vi "PicoScope5000aSetDataBuffers.vi"(5 "enabled array":i16[](array[numeric]), 7 "Buffer and Transfer Settings":T3={"startIndex"=0, "Samples"=1000, "Down Sample Ratio"=1, "Down-Sample Mode"=1} {"Down-Sample Mode" items=["RAW none"=2147483648, "None"=0, "Aggregate"=1, "Decimate"=2, "Average"=4]; "Down Sample Ratio" step=1; "Samples" format="%_6p"}, 8 "error in (no error)":errorcluster, 9 "Device Info":T1={"Driver Version"="2.1.104.3324", "USB Version"="2.0", "Hardware"="1", "Variant"="5244A", "Batch and Serial"="CQ178/007", "Cal Date"="11Jun13", "Kernel Version"="1.0", "Digital HW Version"="1", "Analogue HW Version"="1", "MSO"=FALSE, "Number of channels"=2}, 10 "Data Pointers In":T2, 11 "handle in":i16) -> (0 "error out":errorcluster, 3 "handle out":i16)   [LabVIEW 2010]
doc: "Calls ps5000aSetDataBuffers, and assigns Pico buffers"
uses:
  ps5000a.dll
  shared/PicoBuffers.ctl
  shared/Buffer and Transfer Settings.ctl
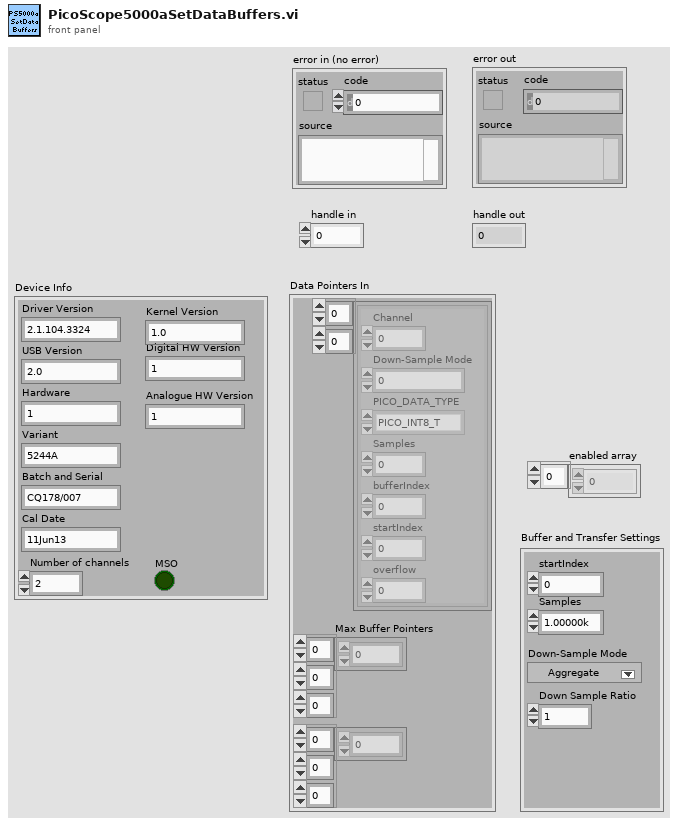
[diagram p1: front panel]
types:
  T1 = cluster{"Driver Version":string, "USB Version":string, "Hardware":string, "Variant":string, "Batch and Serial":string, "Cal Date":string, "Kernel Version":string, "Digital HW Version":string, "Analogue HW Version":string, "MSO":bool, "Number of channels":i16}
  T2 = typedef "PicoBuffers.ctl" = cluster{"Max Buffer Pointers":u64[][][], "Min Buffer Pointers":u64[][][], "StreamingDataInfo":cluster{"Channel":u32, "Down-Sample Mode":u32, "PICO_DATA_TYPE":enum32{"PICO_INT8_T", "PICO_INT16_T", "PICO_INT32_T", "PICO_UINT32_T", "PICO_INT64_T", ""}, "Samples":i32, "bufferIndex":u64, "startIndex":i32, "overflow":i16}[][]}
  T3 = typedef "Buffer and Transfer Settings.ctl" = cluster{"startIndex":u64, "Samples":u64, "Down Sample Ratio":u64, "Down-Sample Mode":u32}
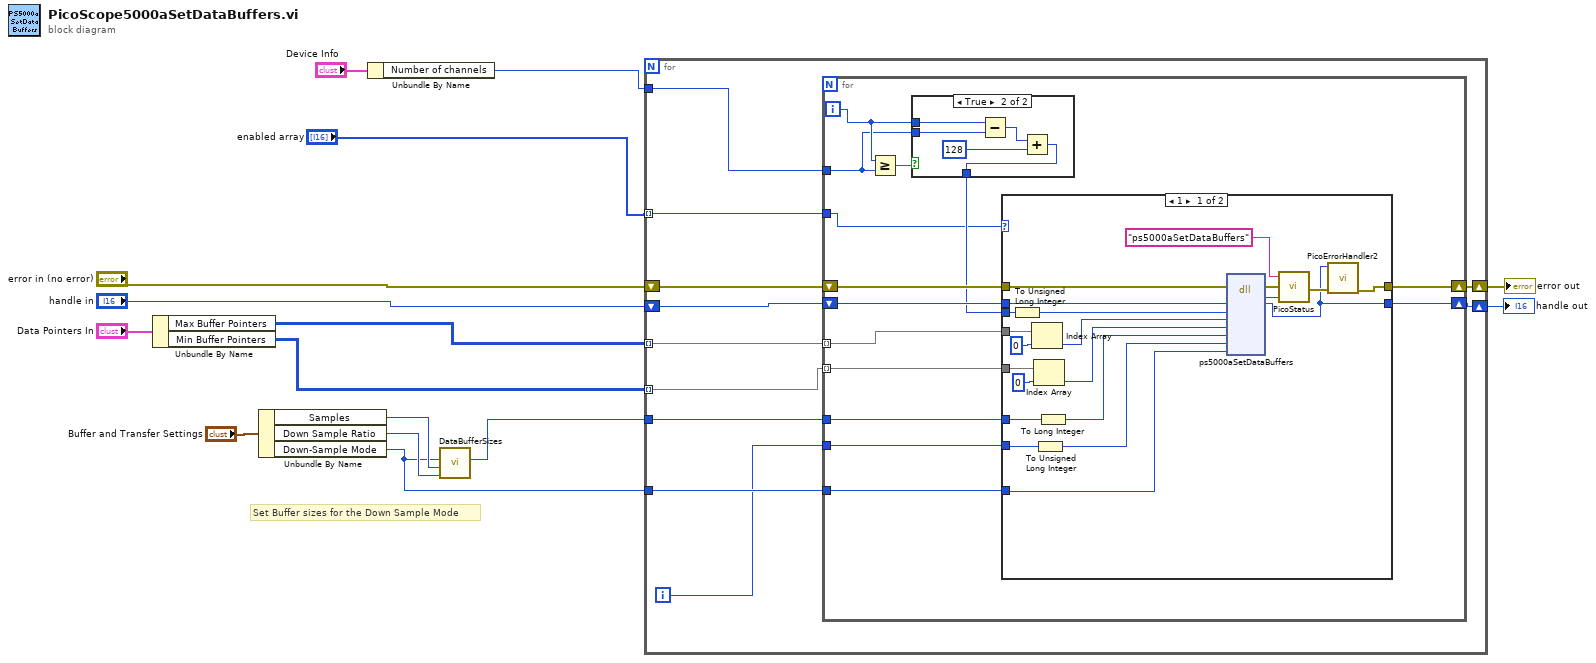
[diagram p0: block diagram]
diagram:
  # "Set Buffer sizes for the Down Sample Mode"
  n1 = Unbundle By Name("Data Pointers In") -> ("Max Buffer Pointers"=w7:u64[][][], "Min Buffer Pointers"=w6:u64[][][])
  n2 = Unbundle By Name("Buffer and Transfer Settings") -> ("Samples"=w9:u64, "Down Sample Ratio"=w10:u64, "Down-Sample Mode"=w8:u32)
  n3 = Unbundle By Name("Device Info") -> ("Number of channels"=w3:i16)
  n4 = call "DataBufferSizes.vi"("Down Sample Ratio"=w10, "Number of Samples"=w9, "Down-Sample Mode"=w8) -> ("Max Buffer Size"=w11:i32)  [unwired: 7 in, 1 out]
  n5 = for {
    tunnel: w11 -> [w22]
    tunnel: w8 -> [w21]
    tunnel: w7 -> [w20] mode=indexing
    tunnel: w6 -> [w19] mode=indexing
    shift-right: [w26] -> w14
    shift-left: "error in (no error)" -> [w24]
    shift-right: [w25] -> w13
    shift-left: "handle in" -> [w23]
    tunnel: w3 -> [w17]
    tunnel: "enabled array" -> [w16] mode=indexing
    i -> [w18]
    n6 = for {
      tunnel: w21 -> [w40]
      tunnel: w22 -> [w37]
      tunnel: w16 -> [w27]
      tunnel: w20 -> [w36] mode=indexing
      shift-right: [w35] -> w26
      shift-left: w24 -> [w39]
      tunnel: w19 -> [w34] mode=indexing
      shift-right: [w33] -> w25
      shift-left: w23 -> [w38]
      tunnel: w18 -> [w32]
      tunnel: w17 -> [w29]
      i -> [w30]
      n7 = Greater Or Equal?(x=w30, y=w29) -> (x >= y?=w31:bool)
      n8 = case shown="True" w31 {
        tunnel: [w41 w45] -> w28
        tunnel: w30 -> [w41 w43]
        tunnel: w29 -> [_ w42]
        frame False {
        }
        frame True {
          n9 = Subtract(x=w43, y=w42) -> (x-y=w44:i32)
          n10 = Add(x=w44, y=128) -> (x+y=w45:i32)
        }
      }
      n11 = case shown="1" w27 {
        tunnel: w28 -> [w57 _]
        tunnel: w39 -> [w67 w69]
        tunnel: w38 -> [w64 w68]
        tunnel: w40 -> [w49 _]
        tunnel: [w61 w69] -> w35
        tunnel: [w60 w68] -> w33
        tunnel: w37 -> [w59 _]
        tunnel: w36 -> [w53 _]
        tunnel: w34 -> [w50 _]
        tunnel: w32 -> [w48 _]
        frame 1 {
          n12 = To Unsigned Long Integer(number=w57) -> (unsigned 32bit integer=w56:u32)
          n13 = Index Array(array=w53, index=0) -> (element=w54:u64)
          n14 = Index Array(array=w50, index=0) -> (element=w51:u64)
          n15 = To Unsigned Long Integer(number=w48) -> (unsigned 32bit integer=w47:u32)
          n16 = To Long Integer(number=w59) -> (32bit integer=w58:i32)
          n17 = dll-call lib="ps5000a.dll" fn="ps5000aSetDataBuffers" ("ps3000.dll:_ps3000_open_unit@0")(error in=w67, "handle"=w64, "channel"=w56, "bufferMax"=w54, "bufferMin"=w51, "bufferLth"=w58, "segmentIndex"=w47, "downSampleRatioMode"=w49) -> (error out=w66:errorcluster, "PICO_STATUS"=w65:u32, "handle"=w60:i16)  [unwired: 8 in, 1 out]
          n18 = call "PicoStatus.vi"("PICO STATUS"=w65, "error in"=w66, "source"="ps5000aSetDataBuffers") -> ("error out"=w62:errorcluster)
          n19 = call "PicoErrorHandler2.vi"("error in (no error)"=w62, "handle In"=w60) -> ("error out"=w61:errorcluster)  [unwired: 9 in]
        }
        frame 0, Default {
        }
      }
    }
  }
  "error out" <- w14
  "handle out" <- w13
